vi "Configure Sweep.vi"(5 "Sweep Time Interval (0.00000512)":dbl=5.12e-06, 7 "Sweep Points (3255)":u32=3255, 8 "error in (no error)":errorcluster, 9 "Sweep Point Offset (0)":dbl, 10 "Power Line Cycles (1)":dbl=1.0, 11 "VISA resource name":refnum<visa-resource-name>) -> (0 "error out":errorcluster, 3 "VISA resource name out":refnum<visa-resource-name>)   [LabVIEW 2019, in "Agilent N7976A.lvlib"]
doc: "Configures sweep options for the power supply.\n\nNote: This VI is only valid on N7900 series."
uses:
  <instrlib>/Agilent N7976A/Agilent N7976A.lvlib
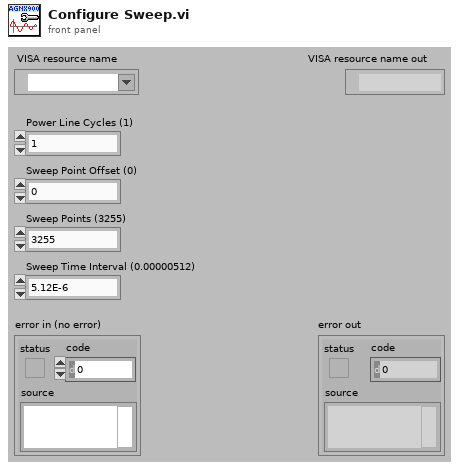
[diagram p1: front panel]
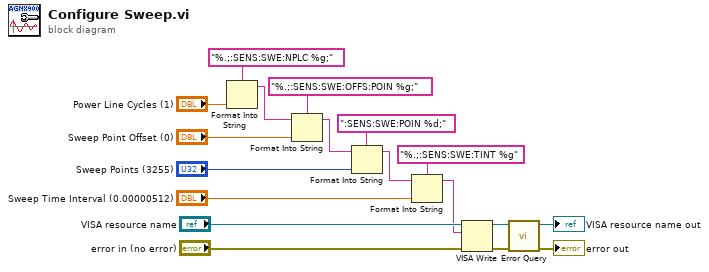
[diagram p0: block diagram]
diagram:
  n1 = Format Into String(format string="%.;:SENS:SWE:NPLC %g;", "Power Line Cycles (1)") -> (resulting string=w1:string)  [unwired: 2 in, 1 out]
  n2 = Format Into String(format string="%.;:SENS:SWE:OFFS:POIN %g;", initial string=w1, "Sweep Point Offset (0)") -> (resulting string=w2:string)  [unwired: 1 in, 1 out]
  n3 = Format Into String(format string=":SENS:SWE:POIN %d;", initial string=w2, "Sweep Points (3255)") -> (resulting string=w3:string)  [unwired: 1 in, 1 out]
  n4 = Format Into String(format string="%.;:SENS:SWE:TINT %g", initial string=w3, "Sweep Time Interval (0.00000512)") -> (resulting string=w11:string)  [unwired: 1 in, 1 out]
  n5 = VISA Write(VISA resource name="VISA resource name", write buffer=w11, error in (no error)="error in (no error)") -> (VISA resource name out=w15:refnum<visa-resource-name>, error out=w16:errorcluster)  [unwired: 1 out]
  n6 = call <instrlib>:"Error Query.vi"("error in (no error)"=w16, "VISA resource name"=w15) -> ("error out"=→"error out":errorcluster, "VISA resource name out"=→"VISA resource name out":refnum<visa-resource-name>)  [unwired: 6 in, 2 out]
